vi "SERVER.vi"() -> ()   [LabVIEW 2023]
panel:
  out "SIGNAL":waveform(dbl)(graph)
  in  "DAQ CHANNEL":tag
  out "# OF SAMPLES":dbl
  out "OBSERVATION TIME [s]":dbl
  out "SAMPLING FREQUENCY [Sample/s]":dbl
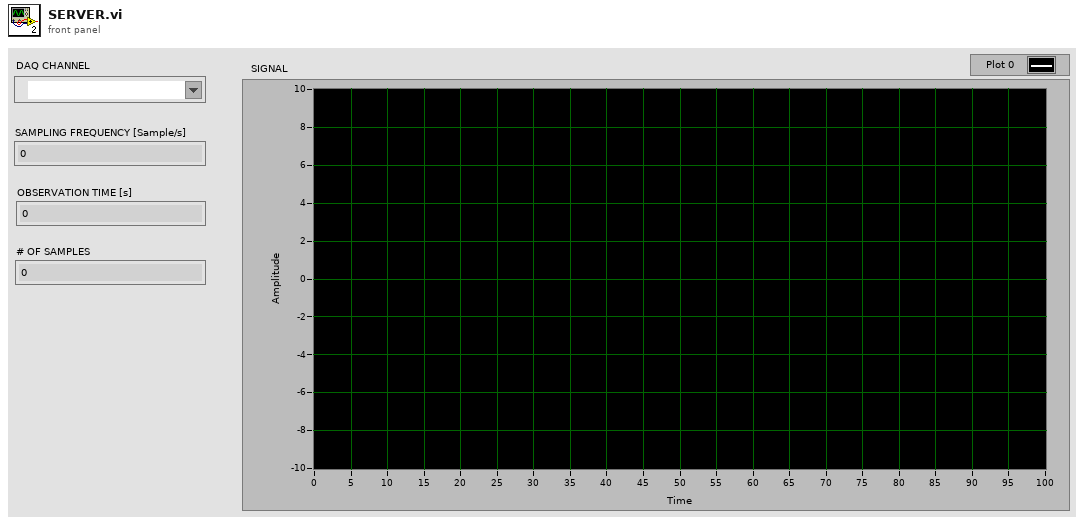
[diagram p1: front panel]
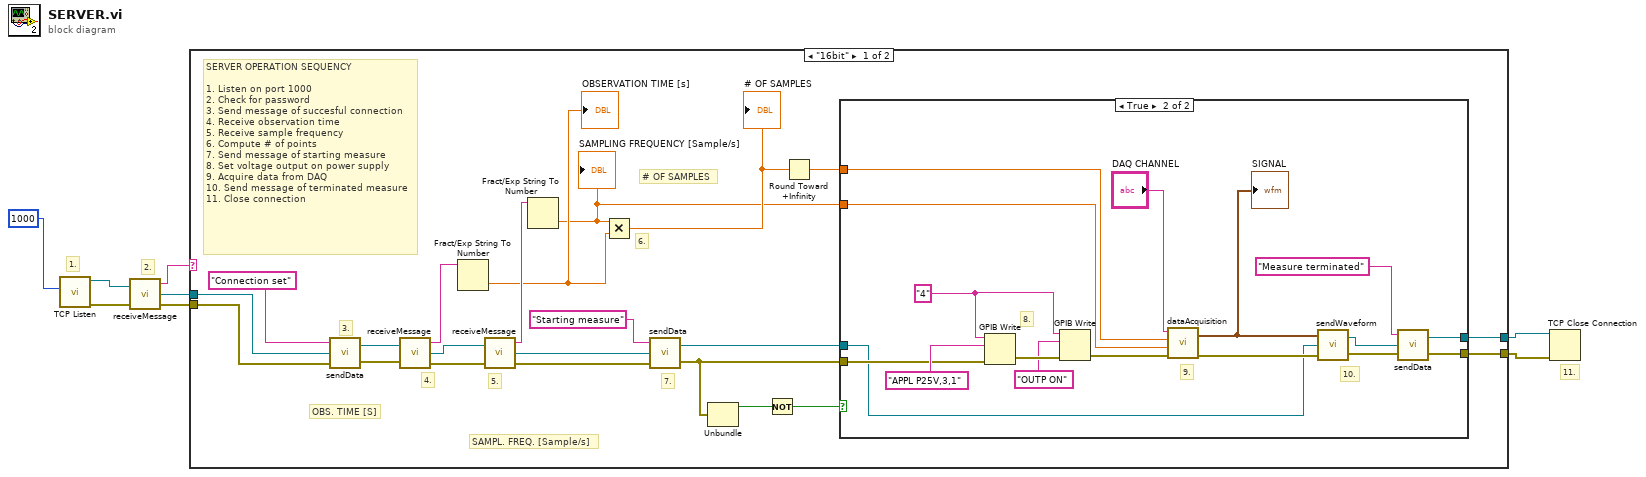
[diagram p0: block diagram]
diagram:
  # "11."
  # "2."
  # "1."
  n1 = call <vilib>:"TCP Listen.vi"("port"=u16 1000) -> ("error out"=w7:errorcluster, "connection ID"=w6:refnum<k5>)  [unwired: 6 in, 3 out]
  n2 = call "receiveMessage.vi"("connection ID"=w6, "error in"=w7) -> ("data out"=w5:string, "connection ID out"=w4:refnum<k5>, "error out"=w3:errorcluster)
  n3 = case shown="\"16bit\"" w5 {
    tunnel: w4 -> [w29 w51]
    tunnel: w3 -> [w30 w50]
    tunnel: [w10 w51] -> w1
    tunnel: [w9 w50] -> w2
    frame "16bit" {
      # "7."
      # "6."
      # "5."
      # "4."
      # "3."
      # "SERVER OPERATION SEQUENCY\n\n1. Listen on port 1000\n2. Check for password\n3. Send message of succesful connection\n4. Receive observation time\n5. Receive sample frequency\n6. Compute # of points\n7. Send message of starting measure\n8. Set voltage output on power supply\n9. Acquire data from DAQ\n10. Send message of terminated measure\n11. Close connection"
      # "# OF SAMPLES"
      # "SAMPL. FREQ. [Sample/s]"
      # "OBS. TIME [S]"
      n4 = call "sendData.vi"("error in"=w30, "connection ID"=w29, "DATA"="Connection set") -> ("error out"=w27:errorcluster, "connection ID out"=w26:refnum<k5>)
      n5 = call "receiveMessage.vi"("connection ID"=w26, "error in"=w27) -> ("data out"=w25:string, "connection ID out"=w24:refnum<k5>, "error out"=w23:errorcluster)
      n6 = Fract/Exp String To Number(string=w25) -> (number=w21:dbl)  [unwired: 3 in, 1 out]
      "OBSERVATION TIME [s]" <- w21
      n7 = call "receiveMessage.vi"("connection ID"=w24, "error in"=w23) -> ("data out"=w22:string, "connection ID out"=w19:refnum<k5>, "error out"=w18:errorcluster)
      n8 = Fract/Exp String To Number(string=w22) -> (number=w11:dbl)  [unwired: 3 in, 1 out]
      "SAMPLING FREQUENCY [Sample/s]" <- w11
      n9 = Multiply(x=w11, y=w21) -> (x*y=w13:dbl)
      "# OF SAMPLES" <- w13
      n10 = call "sendData.vi"("error in"=w18, "connection ID"=w19, "DATA"="Starting measure") -> ("error out"=w16:errorcluster, "connection ID out"=w17:refnum<k5>)
      n11 = Unbundle(w16) -> ("status"=w15:bool)  [unwired: 2 out]
      n12 = Not(x=w15) -> (.not. x?=w14:bool)
      n13 = Round Toward +Infinity(x=w13) -> (ceil(x): smallest int >= x=w12:dbl)
      n14 = case shown="True" w14 {
        tunnel: w16 -> [w32 w48]
        tunnel: w17 -> [w31 w39]
        tunnel: w12 -> [_ w41]
        tunnel: w11 -> [_ w42]
        tunnel: [w32 w34] -> w9
        tunnel: [w31 w33] -> w10
        frame False {
        }
        frame True {
          w46 = "4" ("address string")
          # "10."
          # "9."
          # "8."
          n15 = GPIB Write(0:w46, 1:"APPL P25V,3,1", 3:w48) -> (6:w47:errorcluster)  [unwired: 2 in, 1 out]
          n16 = GPIB Write(0:w46, 1:"OUTP ON", 3:w47) -> (6:w44:errorcluster)  [unwired: 2 in, 1 out]
          n17 = call "dataAcquisition.vi"("error in"=w44, "sampleFrequency"=w42, "samples per channel"=w41, "physical channels"="DAQ CHANNEL") -> ("error out"=w40:errorcluster, "signal"=w38:waveform(dbl))
          "SIGNAL" <- w38
          n18 = call "sendWaveform.vi"("error in"=w40, "connection ID"=w39, "inputSignal"=w38) -> ("error out"=w37:errorcluster, "connection ID out"=w36:refnum<k5>)
          n19 = call "sendData.vi"("error in"=w37, "connection ID"=w36, "DATA"="Measure terminated") -> ("error out"=w34:errorcluster, "connection ID out"=w33:refnum<k5>)
        }
      }
    }
    frame "no", Default {
    }
  }
  n20 = TCP Close Connection(connection ID=w1, error in (no error)=w2) -> ()  [unwired: 1 in, 2 out]
